vi "Close shutter.vi"(8 "error in (no error)":errorcluster, 11 "DAQOrcaFlash in":refnum<class "DAQOrcaFlash.lvclass">) -> (0 "error out":errorcluster, 3 "DAQOrcaFlash out":refnum<class "DAQOrcaFlash.lvclass">)   [LabVIEW 2012, in "DAQOrcaFlash.lvclass"]
uses:
  DAQOrcaFlash.lvclass
  <vilib>/Distrio/Murmex/GenericMessage/GenericMessage.lvclass
  <vilib>/Distrio/Murmex/Murmex/Murmex.lvclass
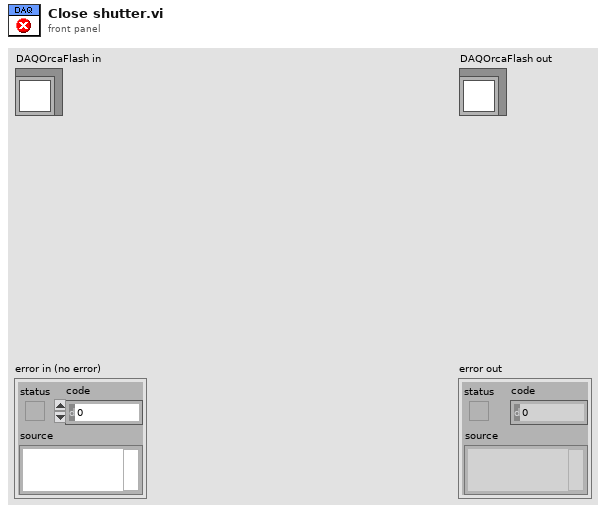
[diagram p1: front panel]
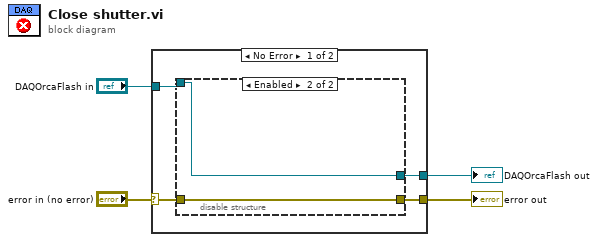
[diagram p0: block diagram]
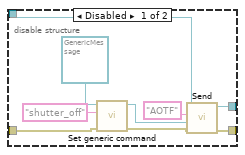
[diagram p2: hidden frame]
diagram:
  n1 = case shown="No Error" "error in (no error)" {
    selector: "error in (no error)" -> [w8 w21]
    tunnel: [w7 w21] -> w3
    tunnel: [w5 w20] -> w1
    tunnel: "DAQOrcaFlash in" -> [w6 w20]
    frame No Error {
      n2 = disable-structure shown="Enabled" {
        disable-tunnel: w8 -> [w16 w18]
        disable-tunnel: [w13 w18] -> w7
        disable-tunnel: w6 -> [w12 w19]
        disable-tunnel: [w11 w19] -> w5
        frame Disabled {
          n3 = call <vilib>:"Set generic command.vi"("error in (no error)"=w16, "generic command"="shutter_off", "GenericMessage in"=refnum<class "GenericMessage.lvclass"> refnum ("Distrio Murmex 1.5:GenericMessage")) -> ("error out"=w14:errorcluster, "GenericMessage out"=w10:refnum<class "GenericMessage.lvclass">)  [unwired: 7 in]
          n4 = call <vilib>:"Send.vi"("error in (no error)"=w14, "Message"=w10, "recipient"="AOTF", "Murmex in"=w12) -> ("error out"=w13:errorcluster, "Murmex out"=w11:refnum<class "DAQOrcaFlash.lvclass">)  [unwired: 6 in]
        }
        frame Enabled {
        }
      }
    }
    frame Error {
    }
  }
  "error out" <- w3
  "DAQOrcaFlash out" <- w1
